vi "PS35_LogFile.vi"(0 "Control unit ID":i32=1 min=1 max=10, 1 "nOpen":i32=1 min=0 max=1, 2 "File name":string="ps35trace.txt", 3 "nAppend":i32 min=0 max=1, 4 "Mode":i32=1 min=0 max=1, 5 "error in (no error)":errorcluster) -> (19 "error out":errorcluster)   [LabVIEW 2020]
doc: "PS35_LogFile.vi, created: 06.03.2009 alex; last change: 22.10.2019 alex;\n\n<B>FUNCTION:</B> \n\nEnable or disable logging.\nThis function offers the possibility to log the interface communication from\nthe software to the control unit (the commands sent from the software and\nthe answers received by the control unit). Two versions are possible, a long\nand a short protocol. The short version contains a head with name of the\ncontrol unit and the starting time, as well as a list of the commands sent and\nthe answers received. The long version also contains the corresponding\ntransmitting and receipting times, and the device status message are displayed\nadditionally. The long version increases the communication time slightly.\n----------------------------------------------------------------------------------------\n<B>INPUT:</B>\n[I32] <B>Control unit ID:</B> control unit index. (Default=1, Range=1...10) \n[I32] <B>nOpen:</B> enable or disable logging. (Default=1, Range=0...1)\n1 - enable logging,\n0 - disable logging.\n[CStr] <B>File name:</B> file name or file path. (Default=\"ps35trace.txt\") \n[I32] <B>nAppend:</B> create or open file. (Default=0, Range=0...1)\n0 - create a new file,\n1 - open an existing file to append.\n[I32] <B>Mode:</B> protocol mode. (Default=1, Range=0...1)\n0 - short protocol (only command and answer strings),\n1 - long protocol (command and answer strings with date and time).\n[CLU] <B>error in</B>\n----------------------------------------------------------------------------------------\n<B>OUTPUT:</B>\n[CLU] <B>error out</B>\n----------------------------------------------------------------------------------------\n<B>SUB-VIs:</B>\n----------------------------------------------------------------------------------------\n<B>EXT-Calls:</B>\nps35.dll (V2.01)\n----------------------------------------------------------------------------------------"
uses:
  ps35.dll
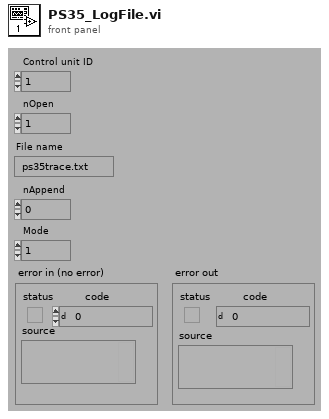
[diagram p1: front panel]
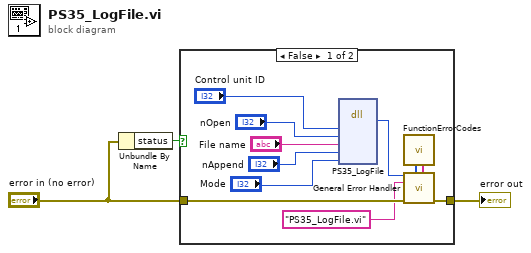
[diagram p0: block diagram]
diagram:
  n1 = Unbundle By Name("error in (no error)") -> ("status"=w1:bool)
  n2 = case shown="False" w1 {
    tunnel: "error in (no error)" -> [w13 w15]
    tunnel: [w12 w15] -> w3
    frame False {
      n3 = dll-call lib="C:/GEECS/Developers Version/source/Device Drivers/OwiSoft/OWISoftOEM/ps35/labview/lv82/ps35.dll" fn="PS35_LogFile"("Index"="Control unit ID", "nOpen"="nOpen", "szFile"="File name", "nAppend"="nAppend", "Mode"="Mode") -> ("Rückgabetyp"=w7:i32)  [unwired: 8 in, 2 out]
      n4 = call "FunctionErrorCodes.vi"() -> ("[user-defined codes]"=w5:i32[], "[user-defined descriptions]"=w4:string[])  [unwired: 8 in]
      n5 = call <vilib>:"General Error Handler.vi"("[error code] (0)"=w7, "[user-defined codes]"=w5, "[user-defined descriptions]"=w4, "[error source] (\" \")"="PS35_LogFile.vi" ("[error source] (\" \")"), "error in (no error)"=w13) -> ("error out"=w12:errorcluster)  [unwired: 6 in, 4 out]
    }
    frame True {
    }
  }
  "error out" <- w3
